vi "PLC_GetVoltage.vi"(4 "Msg":refnum<vi>, 6 "Language":T1, 8 "PLC":refnum<visa-resource-name>, 9 "Selection":T2(ring), 10 "VoltageIO":i32[](array[numeric]), 11 "VISA":refnum<visa-resource-name>) -> (0 "error out":errorcluster, 1 "Array":dbl[](array[numeric]), 3 "VISA resource name out":refnum<visa-resource-name>)   [LabVIEW 2015]
uses:
  CustomControl/Lang_Control.ctl
  PLC_LineOut.vi
panel:
  in  "error in (no error)":errorcluster
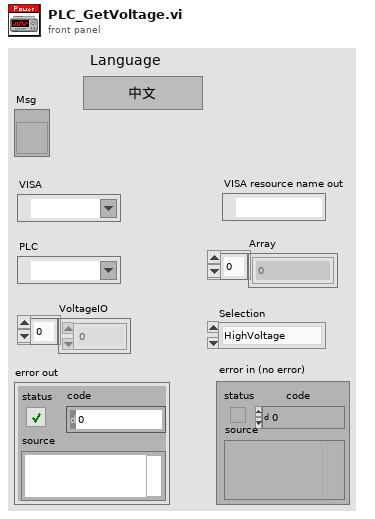
[diagram p1: front panel]
types:
  T1 = typedef "Lang_Control.ctl" = enum16{"中文", "English"}
  T2 = enum16{"HighVoltage", "LowVoltage", "Temperature", "AllOFF"}
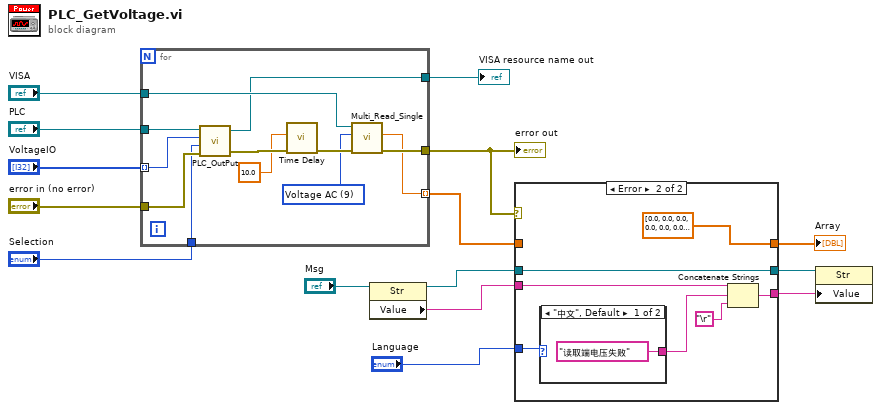
[diagram p0: block diagram]
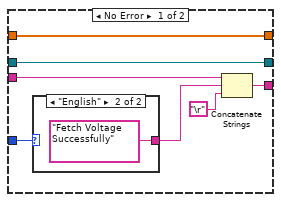
[diagram p2: hidden frame]
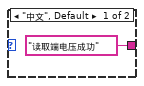
[diagram p3: hidden frame]
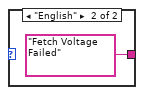
[diagram p4: hidden frame]
diagram:
  n1 = for {
    tunnel: "PLC" -> [w27]
    tunnel: "VISA" -> [w23]
    tunnel: "VoltageIO" -> [w26] mode=indexing
    tunnel: [w25] -> w9
    tunnel: [w24] -> w8 mode=indexing
    tunnel: "error in (no error)" -> [w19]
    tunnel: "Selection" -> [w18]
    tunnel: [w17] -> w10
    w16 = 9 items=["Continuity", "Current AC", "Current DC", "Diode", "Frequency", "Resistance 4-wire", "Period", "Resistance 2-wire", "Temperature", "Voltage AC", "Voltage DC", "Voltage DC Ratio"] ("Measurement Function (10: Voltage DC)")
    n2 = call-poly "PLC_OutPut.vi"("error in (no error)"=w19, "Selection"=w18, "Resistor"=w26, "VISA resource name"=w27) -> ("error out"=w22:errorcluster, "VISA resource name out"=w17:refnum<visa-resource-name>)  [unwired: 1 in]
    n3 = call "Time Delay"("error in (no error)"=w22, "Delay Time (s)"=10.0) -> ("error out"=w21:errorcluster)  [unwired: 9 in]
    n4 = call "Multi_Read_Single.vi"("error in"=w21, "Measurement Function (10: Voltage DC)"=w16, "VISA resource name"=w23) -> ("error out"=w25:errorcluster, "Measurement"=w24:dbl)  [unwired: 7 in]
  }
  "error out" <- w9
  "VISA resource name out" <- w10
  n5 = property class="Str"(reference="Msg") -> (reference out=w5:refnum<vi>, "Value"=w4:string)  [unwired: 1 in, 1 out]
  n6 = case shown="Error" w9 {
    tunnel: w8 -> [w34 _]
    tunnel: [w34 dbl[] [0.0, 0.0, 0.0, 0.0, 0.0, 0.0, 0.0, 0.0, 0.0, 0.0, 0.0, 0.0, 0.0, 0.0, 0.0, 0.0, 0.0, 0.0, 0.0, 0.0]] -> w7
    tunnel: w5 -> [w33 w42]
    tunnel: w4 -> [w32 w39]
    tunnel: [w33 w42] -> w3
    tunnel: [w30 w40] -> w2
    tunnel: "Language" -> [w29 w38]
    frame No Error {
      n7 = case shown="\"English\"" w29 {
        tunnel: ["读取端电压成功" "Fetch Voltage Successfully"] -> w28
        frame "中文", Default {
        }
        frame "English" {
        }
      }
      n8 = Concatenate Strings(w32, w28, "\r") -> (w30:string)
    }
    frame Error {
      n9 = case shown="\"中文\", Default" w38 {
        tunnel: ["读取端电压失败" "Fetch Voltage Failed"] -> w37
        frame "中文", Default {
        }
        frame "English" {
        }
      }
      n10 = Concatenate Strings(w39, w37, "\r") -> (w40:string)
    }
  }
  "Array" <- w7
  n11 = property class="Str"(reference=w3, "Value"=w2) -> ()  [unwired: 1 in, 2 out]
